vi "PID_controller.vi"(2 "Time Period":dbl, 3 "state(k-1)":dbl[](array[numeric]), 4 "Gain":T1, 5 "variable":dbl, 6 "set point":dbl) -> (0 "PID gain":dbl, 1 "state(k)":dbl[](array[numeric]))   [LabVIEW 2019]
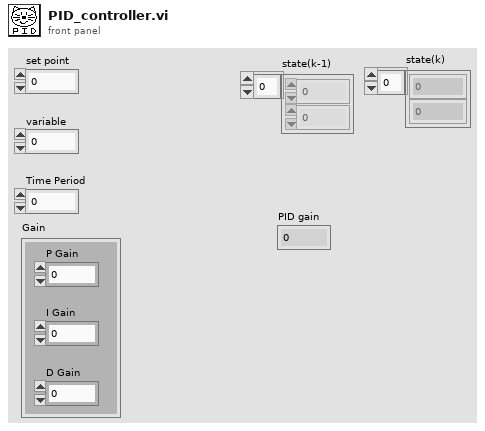
[diagram p1: front panel]
types:
  T1 = cluster{"P Gain":dbl, "I Gain":dbl, "D Gain":dbl}
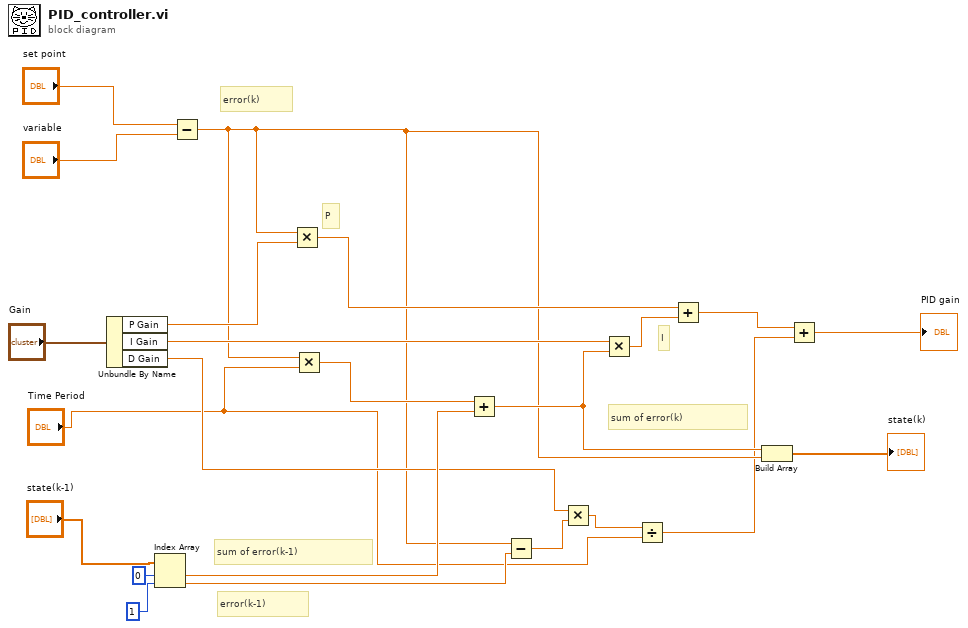
[diagram p0: block diagram]
diagram:
  # "error(k-1)"
  # "sum of error(k-1)"
  # "sum of error(k)"
  # "I"
  # "P"
  # "error(k)"
  n1 = Unbundle By Name("Gain") -> ("P Gain"=w20:dbl, "I Gain"=w18:dbl, "D Gain"=w8:dbl)
  n2 = Index Array(array="state(k-1)", index #1=0 ("index"), index #2=1 ("index")) -> (element #1=w15:dbl, element #2=w10:dbl)
  n3 = Subtract(x="set point", y="variable") -> (x-y=w4:dbl)
  n4 = Multiply(x=w4, y=w20) -> (x*y=w9:dbl)
  n5 = Multiply(x=w4, y="Time Period") -> (x*y=w19:dbl)
  n6 = Add(x=w19, y=w15) -> (x+y=w16:dbl)
  n7 = Subtract(x=w4, y=w10) -> (x-y=w7:dbl)
  n8 = Multiply(x=w8, y=w7) -> (x*y=w2:dbl)
  n9 = Multiply(x=w18, y=w16) -> (x*y=w17:dbl)
  n10 = Divide(x=w2, y="Time Period") -> (x/y=w3:dbl)
  n11 = Add(x=w9, y=w17) -> (x+y=w6:dbl)
  n12 = Build Array(w16, w4) -> (→"state(k)":dbl[])
  n13 = Add(x=w6, y=w3) -> (x+y=→"PID gain":dbl)
